vi "Hexidecimal MAC Address to String.vi"(1 "MAC Address":string) -> (0 "MAC Address (":string)   [LabVIEW 2018]
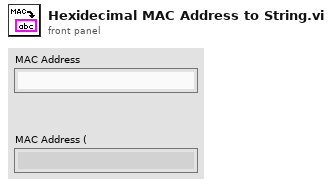
[diagram p1: front panel]
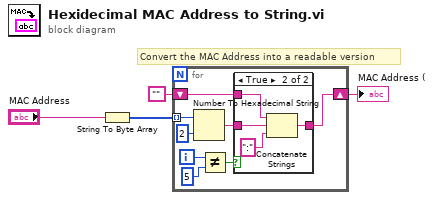
[diagram p0: block diagram]
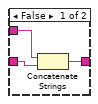
[diagram p2: hidden frame]
diagram:
  # "Convert the MAC Address into a readable version"
  n1 = String To Byte Array(string="MAC Address") -> (unsigned byte array=w4:u8[])
  n2 = for {
    tunnel: w4 -> [w12] mode=indexing
    shift-right: [w11] -> w1
    shift-left: "" -> [w9]
    i -> [w7]
    n3 = Number To Hexadecimal String(1:i16 2 ("width (-)"), 2:w12) -> (0:w10:string)
    n4 = Not Equal?(x=w7, y=5) -> (x != y?=w8:bool)
    n5 = case shown="True" w8 {
      tunnel: [w15 w19] -> w11
      tunnel: w10 -> [w13 w17]
      tunnel: w9 -> [w14 w16]
      frame False {
        n6 = Concatenate Strings(w14, w13) -> (w15:string)
      }
      frame True {
        n7 = Concatenate Strings(w16, w17, ":" ("string")) -> (w19:string)
      }
    }
  }
  "MAC Address (" <- w1
